vi "AOI_Main.vi"() -> ()   [LabVIEW 2017]
uses:
  <vilib>/vision/Image Controls.llb/IMAQ Image.ctl
  <vilib>/userdefined/High Color/IMAQdx.ctl
  <vilib>/vision/driver/IMAQdx.llb/IMAQdx Camera Control Mode.ctl
  <vilib>/Utility/file.llb/Write Delimited Spreadsheet (string).vi
  <vilib>/Utility/file.llb/Read Delimited Spreadsheet (string).vi
  <vilib>/vision/driver/NI_Vision_Acquisition_Software.lvlib
panel:
  out "NG folder array":string[](array[string])
  out "cutting offset\n切割偏移":dbl
  out "damaged\n膠殼破損":dbl
  out "carck\n板裂":dbl
  out "glitch\n毛邊":dbl
  out "number\n數量":dbl
  out "NG code":dbl
  in  "save image\n影像儲存":bool
  in  "output folder\n輸出資料夾":path
  in  "Load setting\n載入參數":bool
  in  "Save setting\n儲存參數":bool
  in  "parameter\n參數":T1={"image imshow (影像繪製)"=FALSE, "side length (mm)\n樣品長度"=0.0, "Main Range (Threshold)\n主輪廓二值化"={"Lower value (上限)"=73.0, "Upper value (下限)"=255.0}, "side velocity threshold\n邊長速度閥值"=0.0, "Sub Range (Threshold)\n次輪廓二值化"={"Lower value (上限)"=73.0, "Upper value (下限)"=255.0}, "close kernel size\n (閉運算核核心大小)"=0.0, "open kernel size\n (開運算核心大小)"=0.0, "side angle offest (threshold)\n邊界角度抑制"=0.0}
  in  "NG_rules( NG規則)":T2
  out "Not DO 2":bool
  out "NG DO 1":bool
  in  "Delay 拍照":u32
  out "img0":T3
  out "Pass DO 0":bool
  out "SOT DI 0":bool
  out "Image\n影像":T3(plugin-control)
  out "TEST.txt Read 2":string[][](array[string])
  out "error Out (no error)":errorcluster
  in  "Exit\n離開":bool
  in  "觸發":bool
  in  "Connect\n連接":bool
  # "Design by OPS Automation Innovation Division"
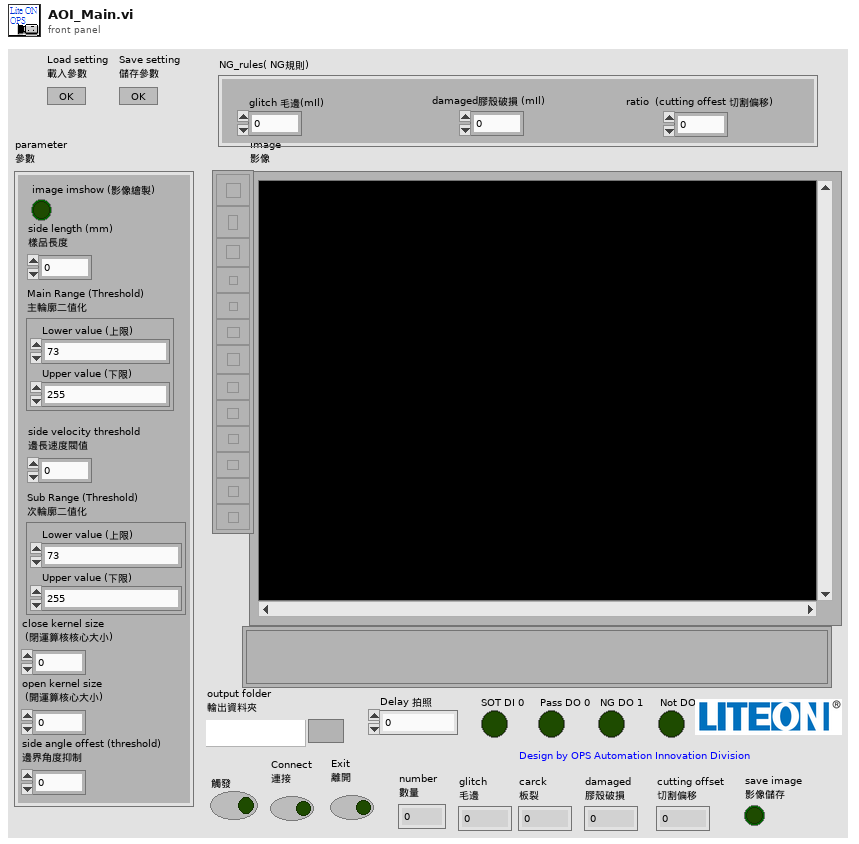
[diagram p1: front panel]
types:
  T1 = cluster{"image imshow (影像繪製)":bool, "side length (mm)\n樣品長度":dbl, "Main Range (Threshold)\n主輪廓二值化":cluster{"Lower value (上限)":sgl, "Upper value (下限)":sgl}, "side velocity threshold\n邊長速度閥值":dbl, "Sub Range (Threshold)\n次輪廓二值化":cluster{"Lower value (上限)":sgl, "Upper value (下限)":sgl}, "close kernel size\n (閉運算核核心大小)":dbl, "open kernel size\n (開運算核心大小)":dbl, "side angle offest (threshold)\n邊界角度抑制":dbl}
  T2 = cluster{"glitch 毛邊(mIl)":dbl, "damaged膠殼破損 (mIl)":dbl, "ratio  (cutting offest 切割偏移)":dbl}
  T3 = typedef "IMAQ Image.ctl" = refnum<image>
  T4 = enum16{"open", "replace", "create", "open or create", "replace or create", "replace or create with confirmation"}
  T5 = typedef "NI_Vision_Acquisition_Software.lvlib/IMAQdx Camera Control Mode.ctl" = enum32{"Controller", "Listener"}
  T6 = typedef "IMAQdx.ctl" = refnum<k21>
  T7 = typedef "Image Type" = u32
  T8 = cluster{"Lower value (上限)":sgl, "Upper value (下限)":sgl}
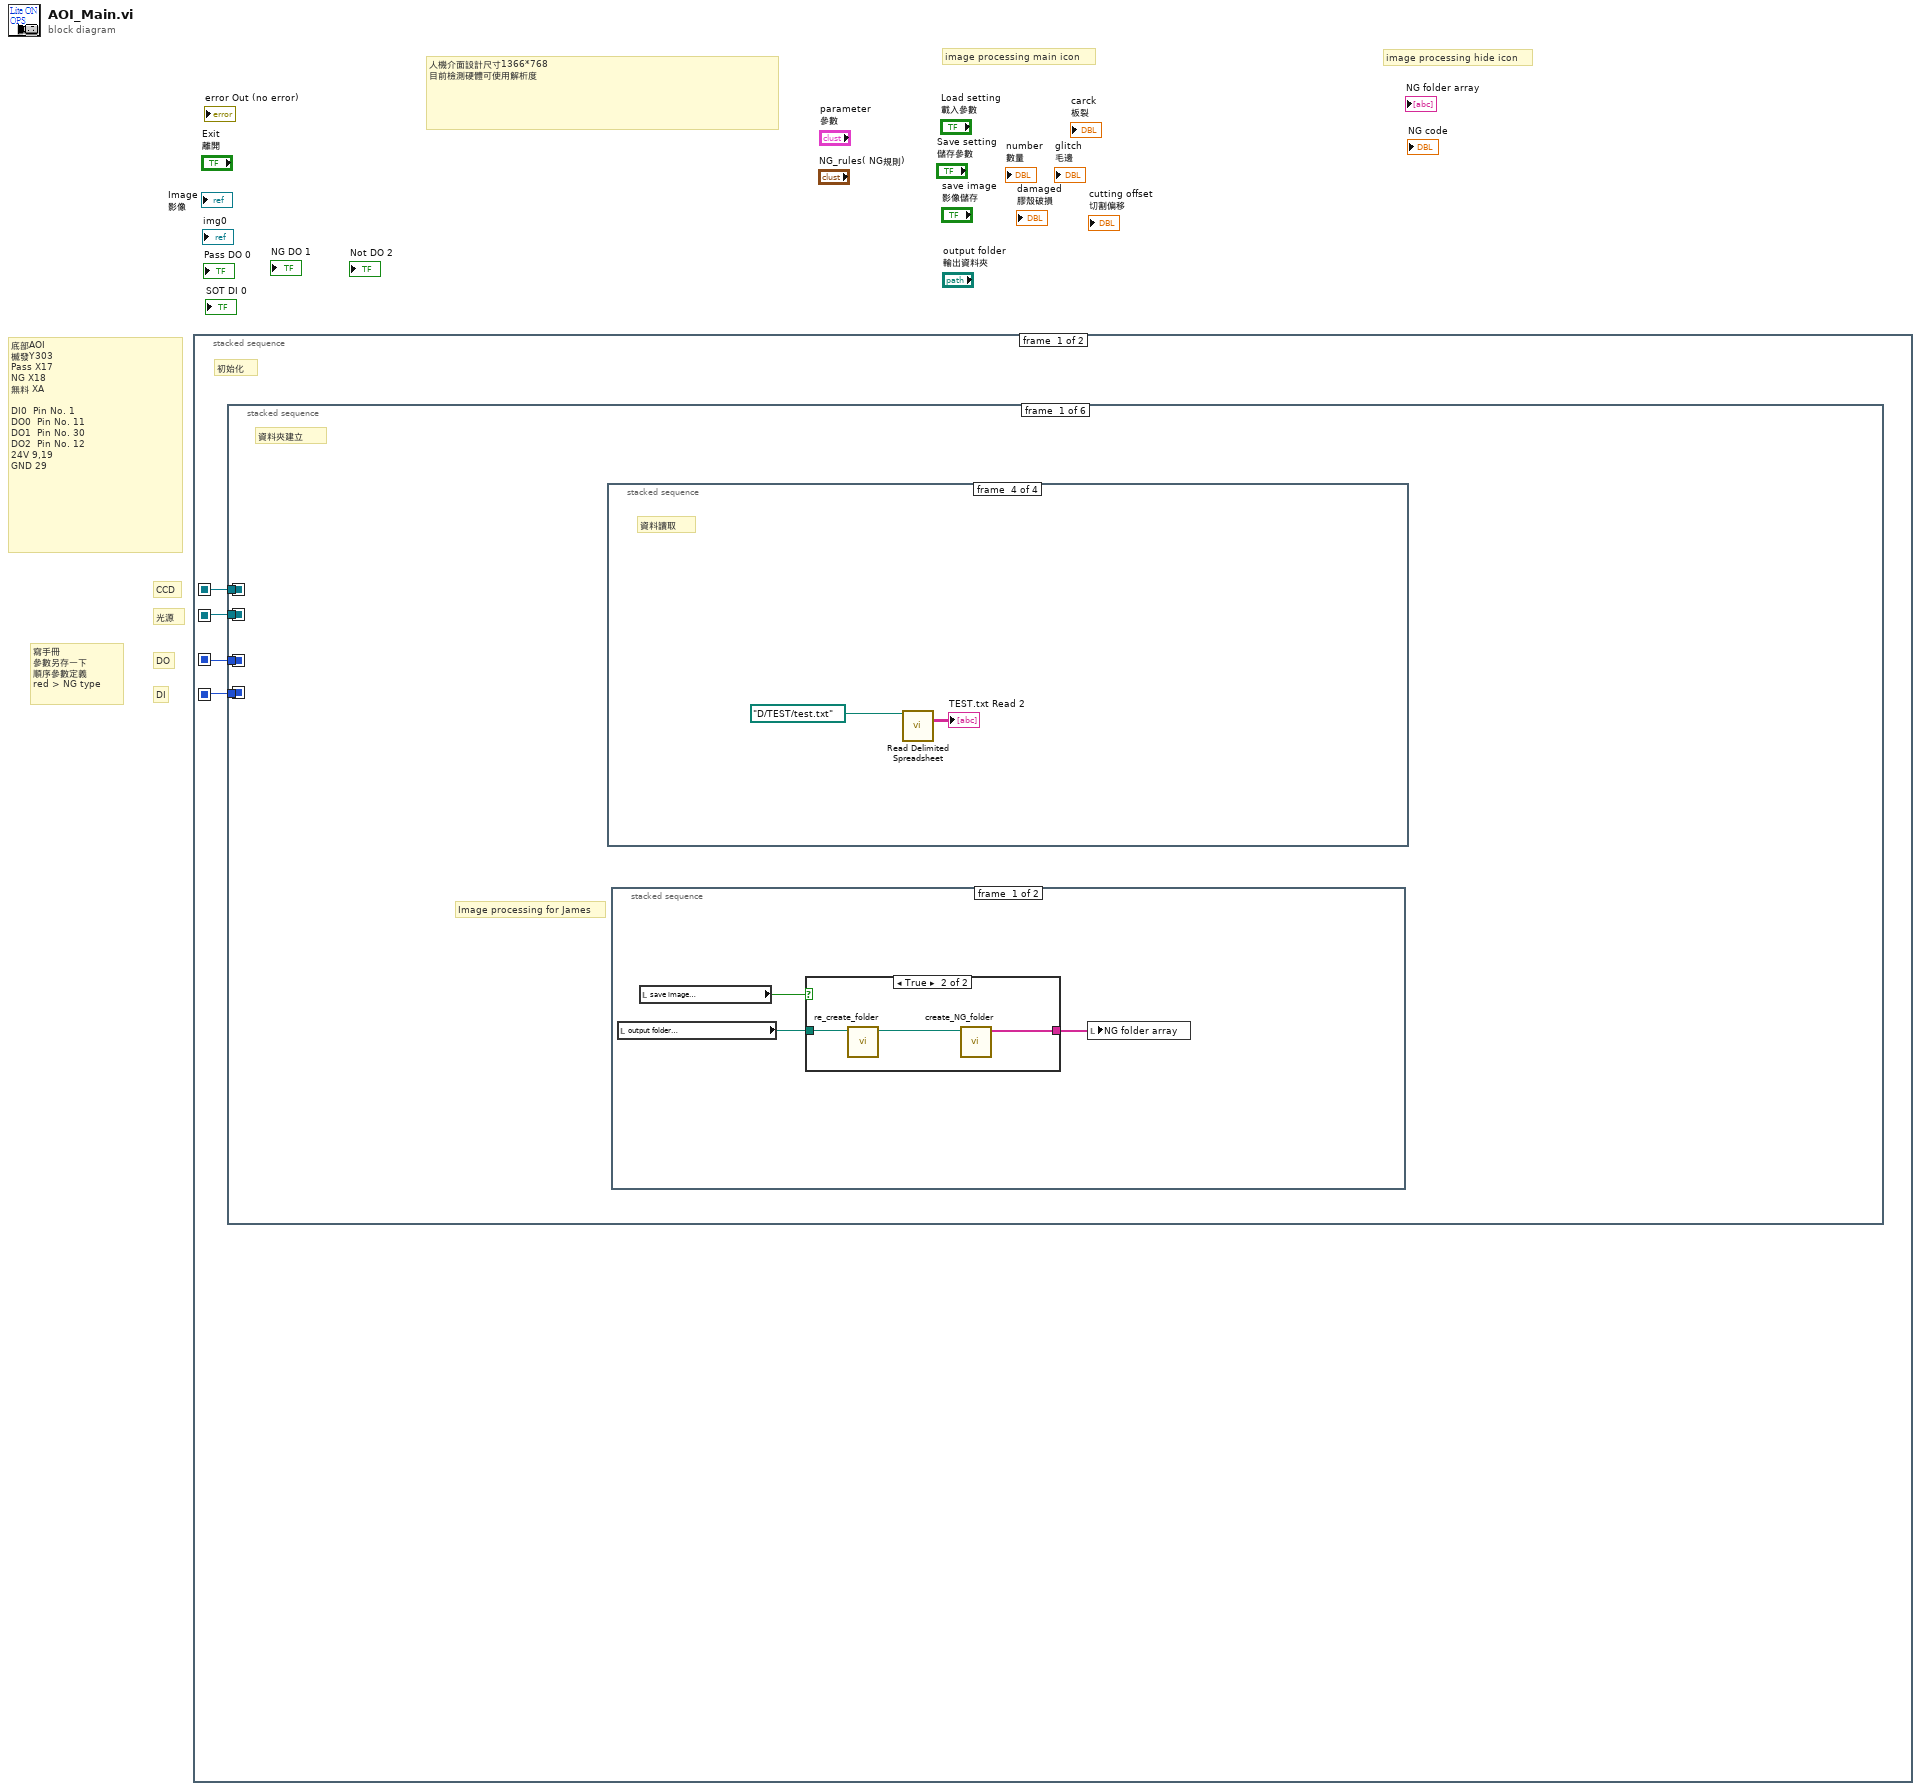
[diagram p0: block diagram]
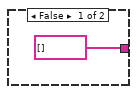
[diagram p2: hidden frame]
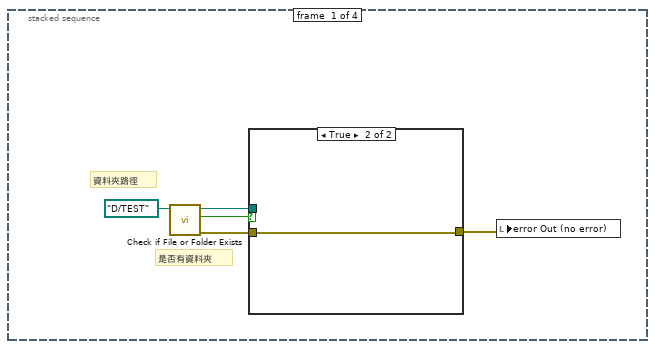
[diagram p4: hidden frame]
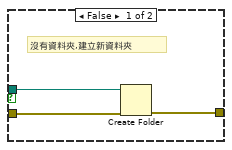
[diagram p5: hidden frame]
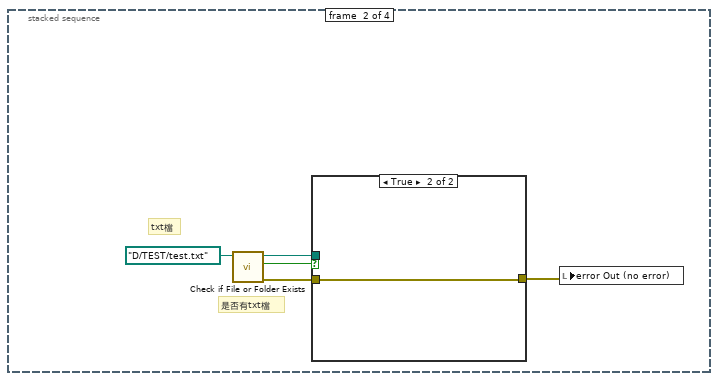
[diagram p6: hidden frame]
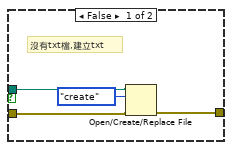
[diagram p7: hidden frame]
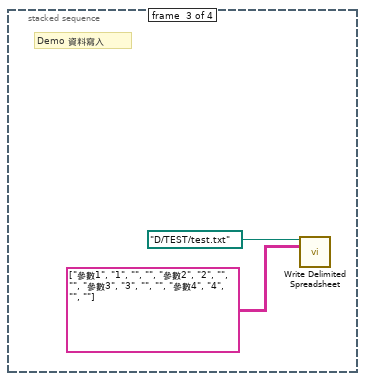
[diagram p8: hidden frame]
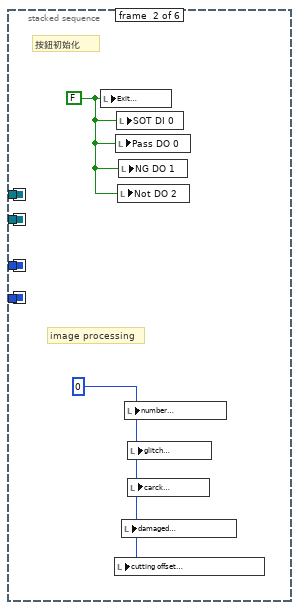
[diagram p9: hidden frame]
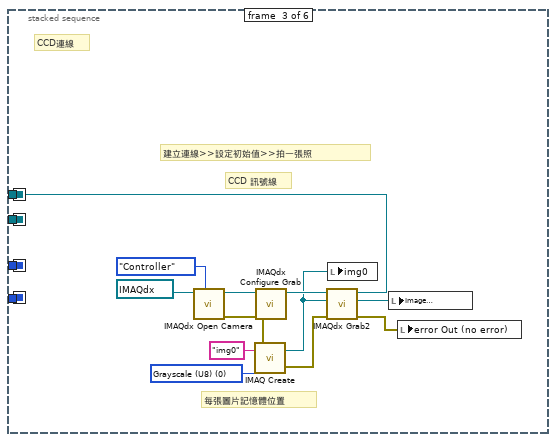
[diagram p10: hidden frame]
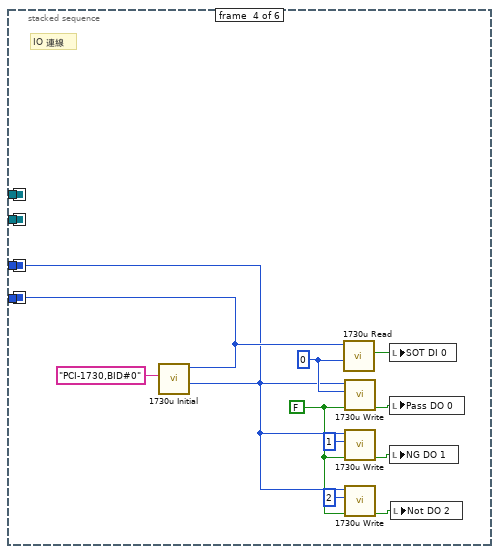
[diagram p11: hidden frame]
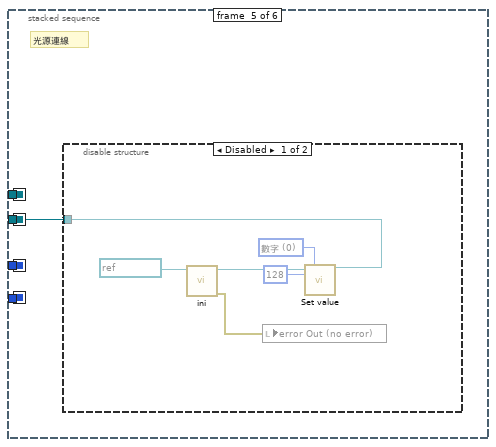
[diagram p12: hidden frame]
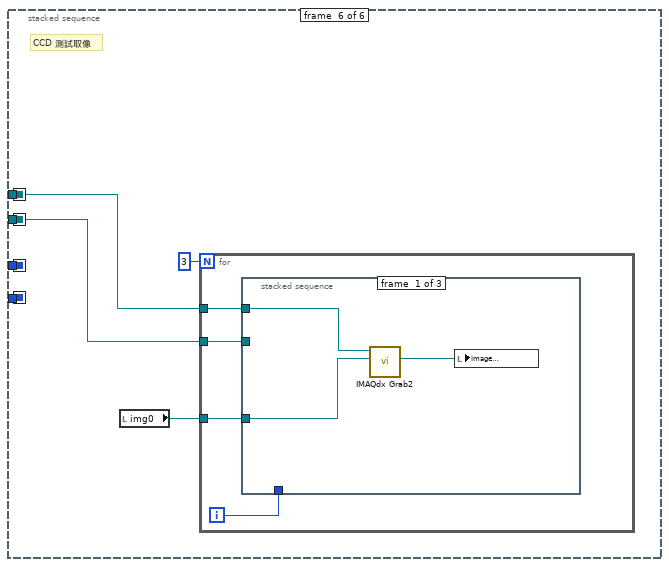
[diagram p14: hidden frame]
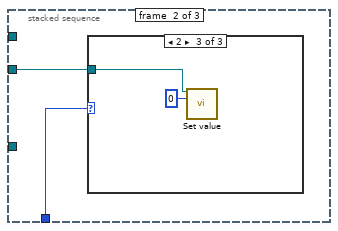
[diagram p15: hidden frame]
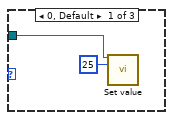
[diagram p16: hidden frame]
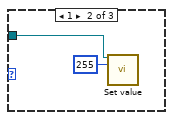
[diagram p17: hidden frame]
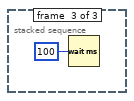
[diagram p18: hidden frame]
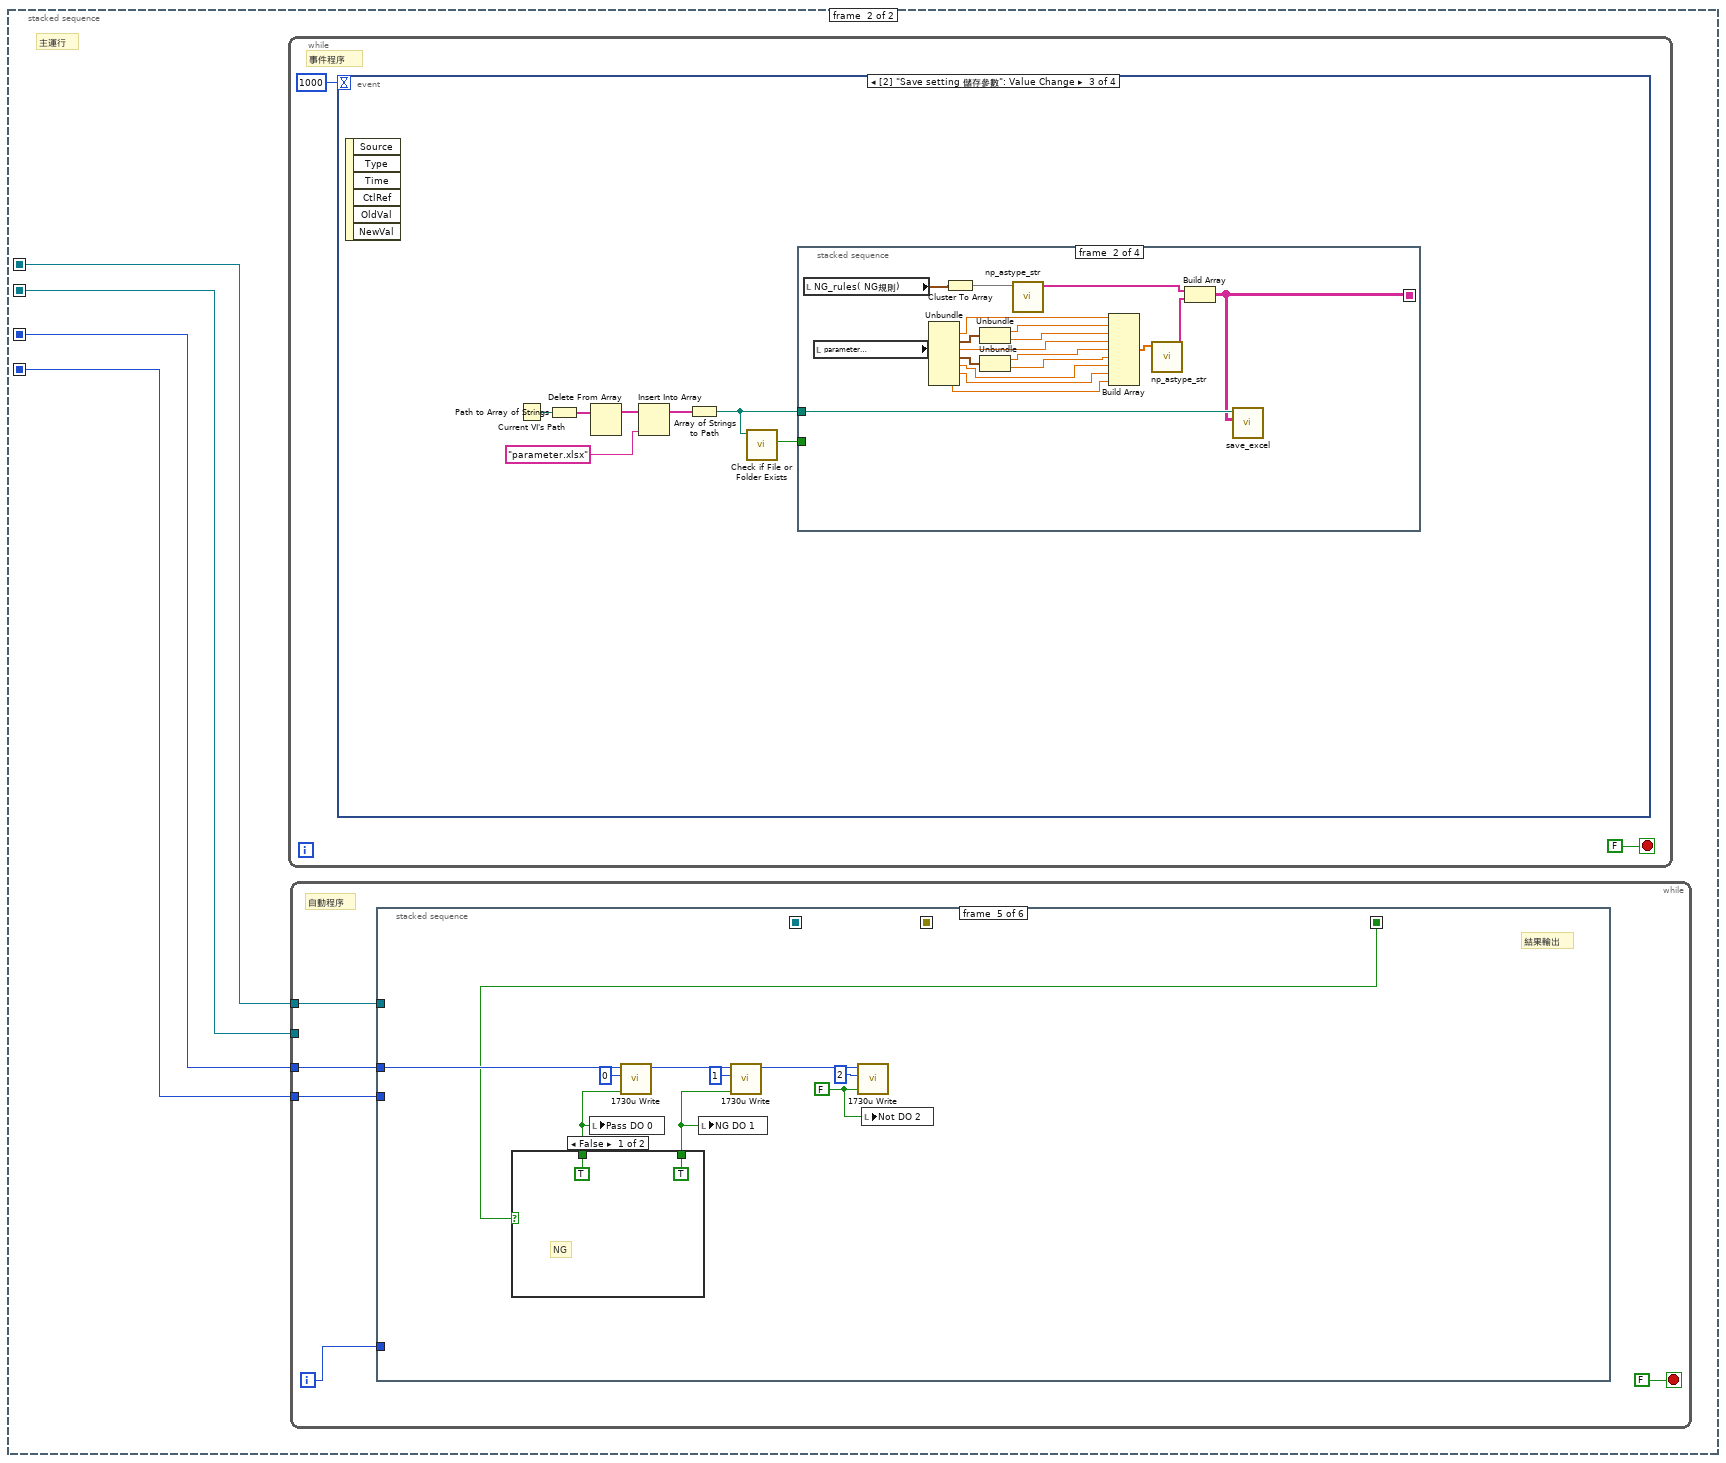
[diagram p19: hidden frame]
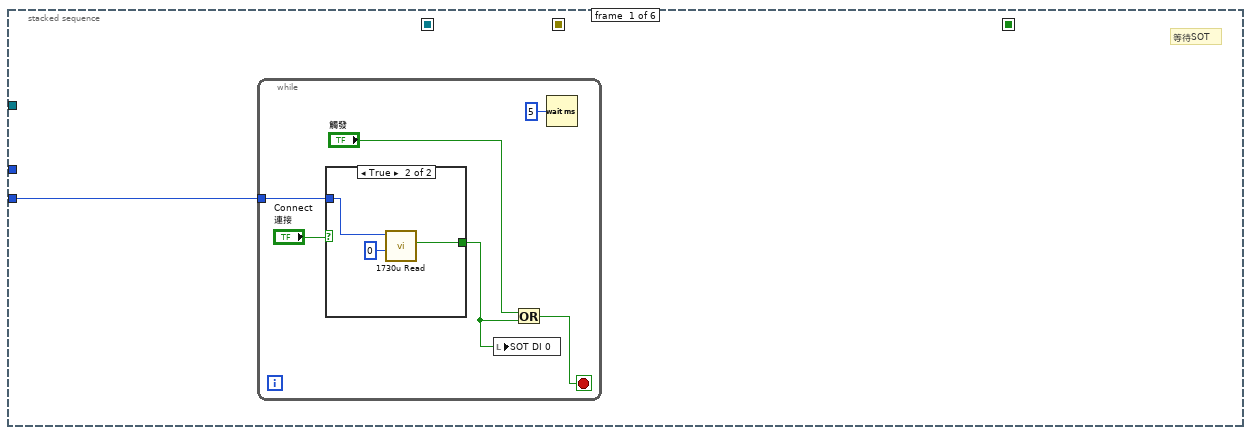
[diagram p20: hidden frame]
diagram:
  # "人機介面設計尺寸1366*768\n目前檢測硬體可使用解析度"
  # "image processing hide icon"
  # "image processing main icon"
  # "寫手冊\n參數另存一下\n順序參數定義\nred > NG type"
  # "底部AOI\n槭發Y303\nPass X17\nNG X18\n無料 XA\n\nDI0  Pin No. 1\nDO0  Pin No. 11\nDO1  Pin No. 30\nDO2  Pin No. 12\n24V 9,19\nGND 29"
  # "DI"
  # "DO"
  # "光源"
  # "CCD"
  n1 = stacked-sequence {
    seq-local: [w4 _] -> [_ w88]
    seq-local: [w3 _] -> [_ w87]
    seq-local: [w2 _] -> [_ w86]
    seq-local: [w1 _] -> [_ w85]
    frame #0 {
      # "初始化"
      n2 = stacked-sequence {
        seq-local: [_ _ w44 _ _ _] -> [_ _ _ _ _ w68]
        seq-local: [_ _ _ _ w58 _] -> [_ _ _ _ _ w67]
        seq-local: [_ _ _ w55 _ _] -> [_ _ _ _ _ _]
        seq-local: [_ _ _ w53 _ _] -> [_ _ _ _ _ _]
        tunnel: [_ _ w44 _ _ _] -> w4
        tunnel: [_ _ _ _ w58 _] -> w3
        tunnel: [_ _ _ w53 _ _] -> w2
        tunnel: [_ _ _ w55 _ _] -> w1
        frame #0 {
          # "Image processing for James"
          # "資料夾建立"
          n3 = stacked-sequence {
            frame #0 {
              # "是否有資料夾"
              # "資料夾路徑"
              n4 = call <vilib>:"Check if File or Folder Exists.vi"("path"=path "D:/TEST") -> ("error out"=w13:errorcluster, "file or folder exists?"=w15:bool, "dup path"=w14:path)  [unwired: 8 in]
              n5 = case shown="True" w15 {
                tunnel: w14 -> [w19 _]
                tunnel: w13 -> [w18 w20]
                tunnel: [w17 w20] -> w12
                frame False {
                  # "沒有資料夾,建立新資料夾"
                  n6 = Create Folder(path (use dialog)=w19, error in=w18) -> (error out=w17:errorcluster)  [unwired: 1 in, 2 out]
                }
                frame True {
                }
              }
              n7 = local write "error Out (no error)"(w12) -> ()
            }
            frame #1 {
              # "是否有txt檔"
              # "txt檔"
              n8 = call <vilib>:"Check if File or Folder Exists.vi"("path"=path "D:/TEST/test.txt") -> ("error out"=w23:errorcluster, "file or folder exists?"=w25:bool, "dup path"=w24:path)  [unwired: 8 in]
              n9 = case shown="True" w25 {
                tunnel: w24 -> [w29 _]
                tunnel: w23 -> [w28 w30]
                tunnel: [w27 w30] -> w22
                frame False {
                  # "沒有txt檔,建立txt"
                  n10 = Open/Create/Replace File(file path (use dialog)=w29, error in=w28, operation (0:open)=T4."create") -> (error out=w27:errorcluster)  [unwired: 3 in, 2 out]
                }
                frame True {
                }
              }
              n11 = local write "error Out (no error)"(w22) -> ()
            }
            frame #2 {
              # "Demo 資料寫入"
              n12 = call-poly <vilib>:"Write Delimited Spreadsheet.vi"("file path (dialog if empty)"=path "D:/TEST/test.txt" ("path"), "2D data"=string[][] [["參數1", "1", "", ""], ["參數2", "2", "", ""], ["參數3", "3", "", ""], ["參數4", "4", "", ""]]) -> ()  [unwired: 12 in, 2 out]
            }
            frame #3 {
              # "資料讀取"
              n13 = call-poly <vilib>:"Read Delimited Spreadsheet.vi"("file path (dialog if empty)"=path "D:/TEST/test.txt" ("path")) -> ("all rows"=→"TEST.txt Read 2":string[][])  [unwired: 9 in, 5 out]
            }
          }
          n14 = stacked-sequence {
            frame #0 {
              n15 = local read "output folder\n輸出資料夾"() -> (w7:path)
              n16 = local read "save image\n影像儲存"() -> (w5:bool)
              n17 = case shown="True" w5 {
                tunnel: w7 -> [_ w11]
                tunnel: [string[] [] ("NG folder array") w9] -> w6
                frame False {
                }
                frame True {
                  n18 = call "re_create_folder.vi"("output folder in"=w11) -> ("output folder out"=w10:path)  [unwired: 10 in]
                  n19 = call "create_NG_folder.vi"("output folder in"=w10) -> ("NG folder array"=w9:string[])  [unwired: 10 in]
                }
              }
              n20 = local write "NG folder array"(w6) -> ()
            }
            frame #1 {
            }
          }
        }
        frame #1 {
          w35 = 0
          w36 = FALSE ("Exit")
          # "image processing"
          # "按鈕初始化"
          n21 = local write "Exit\n離開"(w36) -> ()
          n22 = local write "cutting offset\n切割偏移"(w35) -> ()
          n23 = local write "Pass DO 0"(w36) -> ()
          n24 = local write "SOT DI 0"(w36) -> ()
          n25 = local write "Not DO 2"(w36) -> ()
          n26 = local write "NG DO 1"(w36) -> ()
          n27 = local write "damaged\n膠殼破損"(w35) -> ()
          n28 = local write "number\n數量"(w35) -> ()
          n29 = local write "glitch\n毛邊"(w35) -> ()
          n30 = local write "carck\n板裂"(w35) -> ()
        }
        frame #2 {
          w40 = T7 0 items=["Grayscale (U8)", "Grayscale (I16)", "Grayscale (SGL)", "Complex (CSG)", "RGB (U32)", "HSL (U32)", "RGB (U64)", "Grayscale (U16)"] ("Image Type")
          # "每張圖片記憶體位置"
          # "建立連線>>設定初始值>>拍一張照"
          # "CCD 訊號線"
          # "CCD連線"
          n31 = call <vilib>:"IMAQdx Open Camera.vi"("Camera Control Mode"=IMAQdx_Camera_Control_Mode."Controller", "Session In"=T6 "cam0") -> ("error out"=w47:errorcluster, "Session Out"=w48:T6)  [unwired: 8 in]
          n32 = call <vilib>:"IMAQdx Configure Grab.vi"("error in"=w47, "Session In"=w48) -> ("error out"=w43:errorcluster, "Session Out"=w45:T6)  [unwired: 8 in]
          n33 = call "IMAQ Create"("Image Name"="img0", "Image Type"=w40, "error in (no error)"=w43) -> ("New Image"=w37:T3, "error out"=w42:errorcluster)  [unwired: 2 in]
          n34 = call <vilib>:"IMAQdx Grab2.vi"("error in"=w42, "Image In"=w37, "Session In"=w45) -> ("error out"=w38:errorcluster, "Image Out"=w39:T3, "Session Out"=w44:T6)  [unwired: 5 in, 1 out]
          n35 = local write "img0"(w37) -> ()
          n36 = local write "Image\n影像"(w39) -> ()
          n37 = local write "error Out (no error)"(w38) -> ()
        }
        frame #3 {
          w50 = FALSE ("data")
          w56 = 0 ("portBit")
          # "IO 連線"
          n38 = call <userlib>:"1730u Initial.vi"("physical channels"="PCI-1730,BID#0") -> ("task DO 0~7"=w53:i32, "task DI 0~7"=w55:i32)  [unwired: 6 in, 3 out]
          n39 = call <userlib>:"1730u Read.vi"("portBit"=w56, "DI task in"=w55) -> ("data"=w54:bool)  [unwired: 8 in, 1 out]
          n40 = call <userlib>:"1730u Write.vi"("data"=w50, "portBit"=w56, "DO task in"=w53) -> ()  [unwired: 8 in, 1 out]
          n41 = call <userlib>:"1730u Write.vi"("data"=w50, "portBit"=1, "DO task in"=w53) -> ()  [unwired: 8 in, 1 out]
          n42 = call <userlib>:"1730u Write.vi"("data"=w50, "portBit"=2, "DO task in"=w53) -> ()  [unwired: 8 in, 1 out]
          n43 = local write "SOT DI 0"(w54) -> ()
          n44 = local write "Pass DO 0"(w50) -> ()
          n45 = local write "NG DO 1"(w50) -> ()
          n46 = local write "Not DO 2"(w50) -> ()
        }
        frame #4 {
          # "光源連線"
          n47 = disable-structure shown="Disabled" {
            disable-tunnel: [w61 _] -> w58
            frame Disabled {
              w62 = u16 0 items=["數字", "閃頻"] ("CST Ctr mode")
              n48 = call <userlib>:"ini.vi"("VISA resource name"=refnum<visa-resource-name> "COM3") -> ("error out"=w60:errorcluster, "VISA resource name out"=w63:refnum<visa-resource-name>)  [unwired: 9 in]
              n49 = local write "error Out (no error)"(w60) -> ()
              n50 = call <userlib>:"Set value.vi"("VISA resource name"=w63, "CST Ctr mode"=w62, "CH1"=i16 128) -> ("VISA resource name out"=w61:refnum<visa-resource-name>)  [unwired: 12 in]
            }
            frame Enabled {
            }
          }
        }
        frame #5 {
          # "CCD 測試取像"
          n51 = local read "img0"() -> (w65:T3)
          n52 = for {
            N: 3 -> [_]
            tunnel: w68 -> [w72]
            tunnel: w67 -> [w70]
            tunnel: w65 -> [w71]
            i -> [w69]
            n53 = stacked-sequence {
              tunnel: w72 -> [w75 _ _]
              tunnel: w71 -> [w74 _ _]
              tunnel: w70 -> [_ w76 _]
              tunnel: w69 -> [_ w77 _]
              frame #0 {
                n54 = call <vilib>:"IMAQdx Grab2.vi"("Image In"=w74, "Session In"=w75) -> ("Image Out"=w73:T3)  [unwired: 6 in, 3 out]
                n55 = local write "Image\n影像"(w73) -> ()
              }
              frame #1 {
                n56 = case shown="2" w77 {
                  tunnel: w76 -> [w79 w81 w83]
                  frame 0, Default {
                    n57 = call <userlib>:"Set value.vi"("VISA resource name"=w79, "CH1"=i16 25) -> ()  [unwired: 13 in, 1 out]
                  }
                  frame 1 {
                    n58 = call <userlib>:"Set value.vi"("VISA resource name"=w81, "CH1"=i16 255) -> ()  [unwired: 13 in, 1 out]
                  }
                  frame 2 {
                    n59 = call <userlib>:"Set value.vi"("VISA resource name"=w83, "CH1"=i16 0) -> ()  [unwired: 13 in, 1 out]
                  }
                }
              }
              frame #2 {
                n60 = Wait (ms)(milliseconds to wait=u32 100) -> ()  [unwired: 1 out]
              }
            }
          }
        }
      }
    }
    frame #1 {
      # "主運行"
      n61 = while {
        stop <- FALSE stop-if-true
        # "事件程序"
        n62 = event shown="[2] \"Save setting 儲存參數\": Value Change" {
          selector: _ -> [_ _ _ _]
          dyn-events: _ -> [_ _ _ _]
          timeout: 1000 -> [_ _ _ _]
          event Timeout {
            n63 = event-data() -> ()  [unwired: 1 in, 3 out]
          }
          event "Exit\n離開": Value Change {
            n64 = event-data() -> ()  [unwired: 1 in, 6 out]
            n65 = stacked-sequence {
              frame #0 {
                # "初始化設備"
              }
              frame #1 {
                # "關閉 LabVIEW"
                n66 = Quit LabVIEW(quit? (T)=TRUE) -> ()
              }
            }
          }
          event "Save setting\n儲存參數": Value Change {
            n67 = event-data() -> ()  [unwired: 1 in, 6 out]
            n68 = Current VI's Path() -> (path=w208:path)
            n69 = Path to Array of Strings(0:w208) -> (2:w209:string[])  [unwired: 1 out]
            n70 = Delete From Array(array=w209) -> (array with subset deleted=w210:string[])  [unwired: 2 in, 1 out]
            n71 = Insert Into Array(array=w210, new element="parameter.xlsx" ("string")) -> (w211:string[])  [unwired: 1 in]
            n72 = Array of Strings to Path(0:w211) -> (2:w207:path)  [unwired: 1 in]
            n73 = call <vilib>:"Check if File or Folder Exists.vi"("path"=w207) -> ("file or folder exists?"=w206:bool)  [unwired: 8 in, 2 out]
            n74 = stacked-sequence {
              seq-local: [_ w215 _ _] -> [_ _ w243 _]
              tunnel: w207 -> [w213 w220 _ _]
              tunnel: w206 -> [w212 _ _ _]
              frame #0 {
                n75 = case shown="False" w212 {
                  tunnel: w213 -> [_ w214]
                  frame False {
                  }
                  frame True {
                    n76 = Delete(path (use dialog)=w214) -> ()  [unwired: 4 in, 3 out]
                  }
                }
              }
              frame #1 {
                n77 = local read "NG_rules( NG規則)"() -> (w223:T2)
                n78 = local read "parameter\n參數"() -> (w233:T1)
                n79 = Unbundle(w233) -> ("side length (mm)\n樣品長度"=w230:dbl, "Main Range (Threshold)\n主輪廓二值化"=w231:T8, "side velocity threshold\n邊長速度閥值"=w227:dbl, "Sub Range (Threshold)\n次輪廓二值化"=w232:T8, "close kernel size\n (閉運算核核心大小)"=w224:dbl, "open kernel size\n (開運算核心大小)"=w217:dbl, "side angle offest (threshold)\n邊界角度抑制"=w216:dbl)  [unwired: 1 out]
                n80 = Cluster To Array(cluster=w223) -> (array=w222:dbl[])
                n81 = Unbundle(w231) -> ("Lower value (上限)"=w229:sgl, "Upper value (下限)"=w228:sgl)
                n82 = Unbundle(w232) -> ("Lower value (上限)"=w226:sgl, "Upper value (下限)"=w225:sgl)
                n83 = call "np_astype_str.vi"("NG_rules"=w222) -> ("Array"=w221:string[])  [unwired: 10 in]
                n84 = Build Array(w230, w229, w228, w227, w226, w225, w224, w217, w216) -> (w219:dbl[])
                n85 = call "np_astype_str.vi"("NG_rules"=w219) -> ("Array"=w218:string[])  [unwired: 10 in]
                n86 = Build Array(w221, w218) -> (w215:string[][])
                n87 = call "save_excel.vi"("data in"=w215, "Path"=w220) -> ()  [unwired: 10 in]
              }
              frame #2 {
                n88 = call "re_create_folder.vi"("output folder in"=path "C:/userss") -> ("output folder out"=w238:path)  [unwired: 10 in]
                n89 = Path to Array of Strings(0:w238) -> (2:w241:string[])  [unwired: 1 out]
                n90 = Delete From Array(array=w241) -> (array with subset deleted=w240:string[])  [unwired: 2 in, 1 out]
                n91 = Insert Into Array(array=w240, new element="userss" ("string")) -> (w236:string[])  [unwired: 1 in]
                n92 = Insert Into Array(array=w236, new element="parameter.xlsx" ("string")) -> (w235:string[])  [unwired: 1 in]
                n93 = Array of Strings to Path(0:w235) -> (2:w237:path)  [unwired: 1 in]
                n94 = call "save_excel.vi"("data in"=w243, "Path"=w237) -> ()  [unwired: 10 in]
              }
              frame #3 {
                n95 = One Button Dialog(message="Save success!") -> ()  [unwired: 1 in, 1 out]
              }
            }
          }
          event "Load setting\n載入參數": Value Change {
            n96 = event-data() -> ()  [unwired: 1 in, 6 out]
            n97 = Current VI's Path() -> (path=w248:path)
            n98 = Path to Array of Strings(0:w248) -> (2:w249:string[])  [unwired: 1 out]
            n99 = Delete From Array(array=w249) -> (array with subset deleted=w250:string[])  [unwired: 2 in, 1 out]
            n100 = Insert Into Array(array=w250, new element="parameter.xlsx" ("string")) -> (w251:string[])  [unwired: 1 in]
            n101 = Array of Strings to Path(0:w251) -> (2:w247:path)  [unwired: 1 in]
            n102 = call <vilib>:"Check if File or Folder Exists.vi"("path"=w247) -> ("file or folder exists?"=w246:bool)  [unwired: 8 in, 2 out]
            n103 = case shown="True" w246 {
              tunnel: w247 -> [_ w253]
              frame False {
              }
              frame True {
                n104 = call "load_excel.vi"("Path"=w253) -> ("data"=w252:string[][])  [unwired: 10 in]
                n105 = stacked-sequence {
                  tunnel: w252 -> [w262 w301 _]
                  frame #0 {
                    n106 = Index Array(array=w262, index (row)=1) -> (element=w276:string[])  [unwired: 1 in]
                    n107 = Index Array(array=w262, index (row)=1) -> (element=w263:string[])  [unwired: 1 in]
                    n108 = Index Array(array=w262, index (row)=1) -> (element=w269:string[])  [unwired: 1 in]
                    n109 = Index Array(array=w262, index (row)=1) -> (element=w268:string[])  [unwired: 1 in]
                    n110 = Index Array(array=w276, index=2 ("index (row)")) -> (element=w257:string)
                    n111 = Index Array(array=w263, index=1 ("index (row)")) -> (element=w256:string)
                    n112 = Index Array(array=w269, index=4 ("index (row)")) -> (element=w255:string)
                    n113 = Index Array(array=w268, index=5 ("index (row)")) -> (element=w254:string)
                    n114 = Scan From String(input string=w256) -> (output 1=w261:dbl)  [unwired: 4 in, 3 out]
                    n115 = Scan From String(input string=w257) -> (output 1=w260:dbl)  [unwired: 4 in, 3 out]
                    n116 = Scan From String(input string=w255) -> (output 1=w259:dbl)  [unwired: 4 in, 3 out]
                    n117 = Scan From String(input string=w254) -> (output 1=w258:dbl)  [unwired: 4 in, 3 out]
                    n118 = local read "parameter\n參數"() -> (w274:T1)
                    n119 = Bundle By Name(cluster=w274, "Main Range (Threshold)\n主輪廓二值化.Lower value (上限)"=w261, "Main Range (Threshold)\n主輪廓二值化.Upper value (下限)"=w260, "Sub Range (Threshold)\n次輪廓二值化.Lower value (上限)"=w259, "Sub Range (Threshold)\n次輪廓二值化.Upper value (下限)"=w258) -> (w273:T1)
                    n120 = local write "parameter\n參數"(w273) -> ()
                  }
                  frame #1 {
                    n121 = Index Array(array=w301, index (row)=1) -> (element=w277:string[])  [unwired: 1 in]
                    n122 = Index Array(array=w301, index (row)=0) -> (element=w303:string[])  [unwired: 1 in]
                    n123 = Index Array(array=w277, index=8 ("index (row)")) -> (element=w280:string)
                    n124 = Index Array(array=w277, index=7 ("index (row)")) -> (element=w287:string)
                    n125 = Index Array(array=w277, index=6 ("index (row)")) -> (element=w288:string)
                    n126 = Index Array(array=w277, index=3 ("index (row)")) -> (element=w289:string)
                    n127 = Index Array(array=w303, index=1 ("index (row)")) -> (element=w292:string)
                    n128 = Index Array(array=w277, index=0 ("index (row)")) -> (element=w290:string)
                    n129 = Index Array(array=w303, index=0 ("index (row)")) -> (element=w293:string)
                    n130 = Index Array(array=w303, index=2 ("index (row)")) -> (element=w291:string)
                    n131 = Scan From String(input string=w280) -> (output 1=w278:dbl)  [unwired: 4 in, 3 out]
                    n132 = Scan From String(input string=w291) -> (output 1=w285:dbl)  [unwired: 4 in, 3 out]
                    n133 = Scan From String(input string=w287) -> (output 1=w281:dbl)  [unwired: 4 in, 3 out]
                    n134 = Scan From String(input string=w293) -> (output 1=w294:dbl)  [unwired: 4 in, 3 out]
                    n135 = Scan From String(input string=w292) -> (output 1=w286:dbl)  [unwired: 4 in, 3 out]
                    n136 = Scan From String(input string=w290) -> (output 1=w284:dbl)  [unwired: 4 in, 3 out]
                    n137 = Scan From String(input string=w289) -> (output 1=w283:dbl)  [unwired: 4 in, 3 out]
                    n138 = Scan From String(input string=w288) -> (output 1=w282:dbl)  [unwired: 4 in, 3 out]
                    n139 = local read "NG_rules( NG規則)"() -> (w304:T2)
                    n140 = Bundle By Name(cluster=w304, "glitch 毛邊(mIl)"=w294, "damaged膠殼破損 (mIl)"=w286, "ratio  (cutting offest 切割偏移)"=w285) -> (w307:T2)
                    n141 = local read "parameter\n參數"() -> (w295:T1)
                    n142 = Bundle By Name(cluster=w295, "side length (mm)\n樣品長度"=w284, "side velocity threshold\n邊長速度閥值"=w283, "close kernel size\n (閉運算核核心大小)"=w282, "open kernel size\n (開運算核心大小)"=w281, "side angle offest (threshold)\n邊界角度抑制"=w278) -> (w299:T1)
                    n143 = local write "NG_rules( NG規則)"(w307) -> ()
                    n144 = local write "parameter\n參數"(w299) -> ()
                  }
                  frame #2 {
                    n145 = One Button Dialog(message="Save success!") -> ()  [unwired: 1 in, 1 out]
                  }
                }
              }
            }
          }
        }
      }
      n146 = while {
        tunnel: w88 -> [w90]
        tunnel: w87 -> [_]
        tunnel: w86 -> [w91]
        tunnel: w85 -> [w92]
        i -> [w89]
        stop <- FALSE stop-if-true
        # "自動程序"
        n147 = stacked-sequence {
          seq-local: [_ _ w114 _ _ _] -> [_ _ _ w140 _ _]
          seq-local: [_ _ w112 _ _ _] -> [_ _ _ _ _ _]
          seq-local: [_ _ _ w137 _ _] -> [_ _ _ _ w184 _]
          tunnel: w92 -> [w94 _ _ _ _ w201]
          tunnel: w91 -> [_ w111 _ _ w190 _]
          tunnel: w90 -> [_ _ w115 _ _ _]
          tunnel: w89 -> [_ _ _ w129 _ _]
          frame #0 {
            # "等待SOT"
            n148 = while {
              tunnel: w94 -> [w96]
              stop <- w100 stop-if-true
              n149 = case shown="True" "Connect\n連接" {
                tunnel: w96 -> [_ w104]
                tunnel: [FALSE ("data") w102] -> w95
                frame False {
                }
                frame True {
                  n150 = call <userlib>:"1730u Read.vi"("portBit"=0, "DI task in"=w104) -> ("data"=w102:bool)  [unwired: 8 in, 1 out]
                }
              }
              n151 = local write "SOT DI 0"(w95) -> ()
              n152 = Or(x="觸發", y=w95) -> (x .or. y?=w100:bool)
              n153 = Wait (ms)(milliseconds to wait=u32 5) -> ()  [unwired: 1 out]
            }
          }
          frame #1 {
            w105 = FALSE ("data")
            # "EOT 切換\nArray整理"
            n154 = local write "Pass DO 0"(w105) -> ()
            n155 = call <userlib>:"1730u Write.vi"("data"=w105, "portBit"=0, "DO task in"=w111) -> ("DO task out"=w108:i32)  [unwired: 8 in]
            n156 = local write "NG DO 1"(w105) -> ()
            n157 = call <userlib>:"1730u Write.vi"("data"=w105, "portBit"=1, "DO task in"=w108) -> ("DO task out"=w107:i32)  [unwired: 8 in]
            n158 = local write "Not DO 2"(w105) -> ()
            n159 = call <userlib>:"1730u Write.vi"("data"=w105, "portBit"=2, "DO task in"=w107) -> ()  [unwired: 8 in, 1 out]
          }
          frame #2 {
            # "取像"
            n160 = flat-sequence {
              tunnel: w115 -> [w117]
              tunnel: [w117] -> w113
              tunnel: [w119] -> w114
              tunnel: w113 -> [w121]
              tunnel: [w118] -> w112
              frame #0 {
                n161 = Wait (ms)(milliseconds to wait="Delay 拍照") -> ()  [unwired: 1 out]
              }
              frame #1 {
                n162 = local read "img0"() -> (w120:T3)
                n163 = call <vilib>:"IMAQdx Grab2.vi"("Image In"=w120, "Session In"=w121) -> ("error out"=w118:errorcluster, "Image Out"=w119:T3)  [unwired: 6 in, 2 out]
                n164 = local write "Image\n影像"(w119) -> ()
              }
            }
          }
          frame #3 {
            # "結果"
            # "Error"
            # "拍攝圖片"
            # "檢查"
            n165 = local read "parameter\n參數"() -> (w139:T1)
            n166 = local write "number\n數量"(w129) -> ()
            n167 = Number To Decimal String(number=w129) -> (decimal integer string=w132:string)  [unwired: 1 in]
            n168 = local read "NG_rules( NG規則)"() -> (w138:T2)
            n169 = Concatenate Strings("No." ("string"), w132) -> (w127:string)
            n170 = call "image_processing.vi"("NG_rules"=w138, "parameter"=w139, "image"=w140) -> ("PASS"=w137:bool, "NG code"=w125:dbl, "display image"=w123:T3)  [unwired: 6 in]
            n171 = local write "NG code"(w125) -> ()
            n172 = Number To Decimal String(number=w125) -> (decimal integer string=w135:string)  [unwired: 1 in]
            n173 = local read "NG folder array"() -> (w128:string[])
            n174 = Concatenate Strings("_NG_" ("string"), w135) -> (w130:string)
            n175 = Concatenate Strings(w127, w130) -> (w131:string)
            n176 = Index Array(array=w128, index=w125) -> (element=w124:string)
            n177 = local write "Image\n影像"(w123) -> ()
            n178 = Concatenate Strings(w131, ".png" ("string")) -> (w126:string)
            n179 = local read "save image\n影像儲存"() -> (w122:bool)
            n180 = case shown="True" w122 {
              tunnel: w123 -> [_ w145]
              tunnel: w126 -> [_ w144]
              tunnel: w125 -> [_ w141]
              tunnel: w124 -> [_ w143]
              tunnel: w127 -> [_ w142]
              frame False {
              }
              frame True {
                n181 = case shown="4" w141 {
                  tunnel: w145 -> [w150 w159 w163 w171 w178]
                  tunnel: w144 -> [_ w156 w164 w170 w177]
                  tunnel: w143 -> [w149 w153 w160 w167 w174]
                  tunnel: w142 -> [w148 _ _ _ _]
                  frame 0, Default {
                    n182 = Concatenate Strings(w148, ".bmp" ("string")) -> (w146:string)
                    n183 = Concatenate Strings(w149, w146) -> (w151:string)
                    n184 = String To Path(string=w151) -> (path=w152:path)
                    n185 = call-poly "IMAQ Write File 2"("File Path"=w152, "Image"=w150) -> ()  [unwired: 8 in, 2 out]
                  }
                  frame 1 {
                    n186 = local read "glitch\n毛邊"() -> (w155:dbl)
                    n187 = Concatenate Strings(w153, w156) -> (w157:string)
                    n188 = Increment(x=w155) -> (x+1=w154:dbl)
                    n189 = String To Path(string=w157) -> (path=w158:path)
                    n190 = local write "glitch\n毛邊"(w154) -> ()
                    n191 = call-poly "IMAQ Write File 2"("File Path"=w158, "Image"=w159) -> ()  [unwired: 8 in, 2 out]
                  }
                  frame 2 {
                    n192 = local read "carck\n板裂"() -> (w162:dbl)
                    n193 = Concatenate Strings(w160, w164) -> (w165:string)
                    n194 = Increment(x=w162) -> (x+1=w161:dbl)
                    n195 = String To Path(string=w165) -> (path=w166:path)
                    n196 = local write "carck\n板裂"(w161) -> ()
                    n197 = call-poly "IMAQ Write File 2"("File Path"=w166, "Image"=w163) -> ()  [unwired: 8 in, 2 out]
                  }
                  frame 3 {
                    n198 = local read "damaged\n膠殼破損"() -> (w169:dbl)
                    n199 = Concatenate Strings(w167, w170) -> (w172:string)
                    n200 = Increment(x=w169) -> (x+1=w168:dbl)
                    n201 = String To Path(string=w172) -> (path=w173:path)
                    n202 = local write "damaged\n膠殼破損"(w168) -> ()
                    n203 = call-poly "IMAQ Write File 2"("File Path"=w173, "Image"=w171) -> ()  [unwired: 8 in, 2 out]
                  }
                  frame 4 {
                    n204 = local read "cutting offset\n切割偏移"() -> (w176:dbl)
                    n205 = Concatenate Strings(w174, w177) -> (w179:string)
                    n206 = Increment(x=w176) -> (x+1=w175:dbl)
                    n207 = local write "cutting offset\n切割偏移"(w175) -> ()
                    n208 = String To Path(string=w179) -> (path=w180:path)
                    n209 = call-poly "IMAQ Write File 2"("File Path"=w180, "Image"=w178) -> ()  [unwired: 8 in, 2 out]
                  }
                }
              }
            }
          }
          frame #4 {
            w183 = FALSE ("data")
            # "結果輸出"
            n210 = case shown="False" w184 {
              tunnel: [TRUE TRUE] -> w181
              tunnel: [TRUE FALSE] -> w182
              frame False {
                # "NG"
              }
              frame True {
                # "PASS"
              }
            }
            n211 = local write "Pass DO 0"(w181) -> ()
            n212 = call <userlib>:"1730u Write.vi"("data"=w181, "portBit"=0, "DO task in"=w190) -> ("DO task out"=w187:i32)  [unwired: 8 in]
            n213 = local write "NG DO 1"(w182) -> ()
            n214 = call <userlib>:"1730u Write.vi"("data"=w182, "portBit"=1, "DO task in"=w187) -> ("DO task out"=w186:i32)  [unwired: 8 in]
            n215 = call <userlib>:"1730u Write.vi"("data"=w183, "portBit"=2, "DO task in"=w186) -> ()  [unwired: 8 in, 1 out]
            n216 = local write "Not DO 2"(w183) -> ()
          }
          frame #5 {
            # "EOT 結束\n資料整理"
            n217 = Bundle("task DI 0~7"=w201, 0, FALSE) -> (w197:cluster{"task DI 0~7":i32, i32, bool})  [unwired: 1 in]
            n218 = call <userlib>:"Check DI State 1730u.vi"("Time Out"=u32 3000, "Scan time"=u32 2, "Mode"=enum16{"Check One DI", "Check Two DI"}."Check One DI", "1 DI Mode"=w197) -> ()  [unwired: 7 in, 1 out]
          }
        }
      }
    }
  }
